vi "Read and Update Metadata.vi"(8 "error in (no error)":errorcluster, 11 "Update Metadata":bool) -> (0 "error out":errorcluster, 3 "Plugin Info":T1[](array[typedef]))   [LabVIEW 2021, in "CIFPluginLoader.lvclass"]
uses:
  CIFPluginLoader.lvclass
  typedef/trash_Discovered Plugin.ctl
  CIFCore/Common/Typedef/Version.ctl
  typedef/trash_Plugin Metadata.ctl
  CIFUtilities/CIFConfigurationFile/typedef/Location Type.ctl
  CIFUtilities/CIFConfigurationFile/CIF Configuration File Location.vi
  CIFPluginLoader.lvclass/CIFPluginLoader.ctl
  CIFUtilities/CIFConfigurationFile/CIF Configuration File.lvlib
  <vilib>/Utility/config.llb/NI_LVConfig.lvlib
  CIFCore/Common/CIFCoreCommon.lvlib
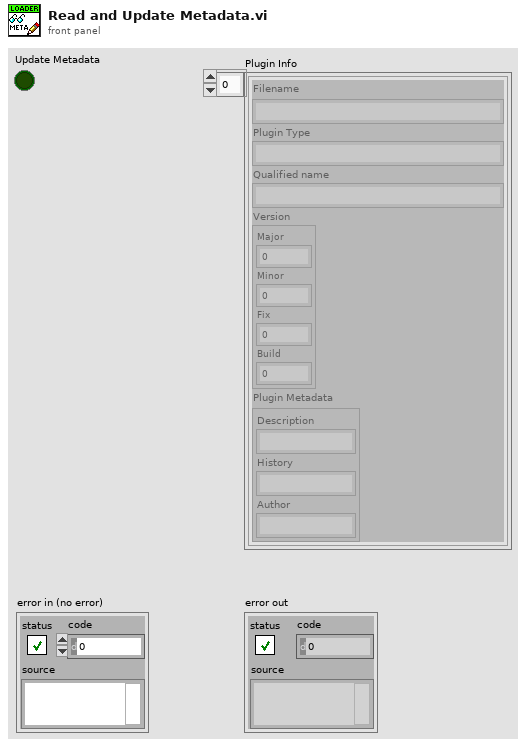
[diagram p1: front panel]
types:
  T1 = typedef "trash_Discovered Plugin.ctl" = cluster{"Filename":string, "Plugin Type":string, "Qualified name":string, "Version":T2, "Plugin Metadata":T3}
  T2 = typedef "CIFCoreCommon.lvlib/Version.ctl" = cluster{"Major":i32, "Minor":i32, "Fix":i32, "Build":i32}
  T3 = typedef "trash_Plugin Metadata.ctl" = cluster{"Description":string, "History":string, "Author":string}
  T4 = typedef "CIF Configuration File.lvlib/Location Type.ctl" = enum16{"Config File", "Manager", "Protos", "Plugins", "UI Plugins", "Logs", "Orchestrations"}
  T5 = typedef "NI_LVConfig.lvlib/Config Data RefNum.ctl" = refnum<k1>
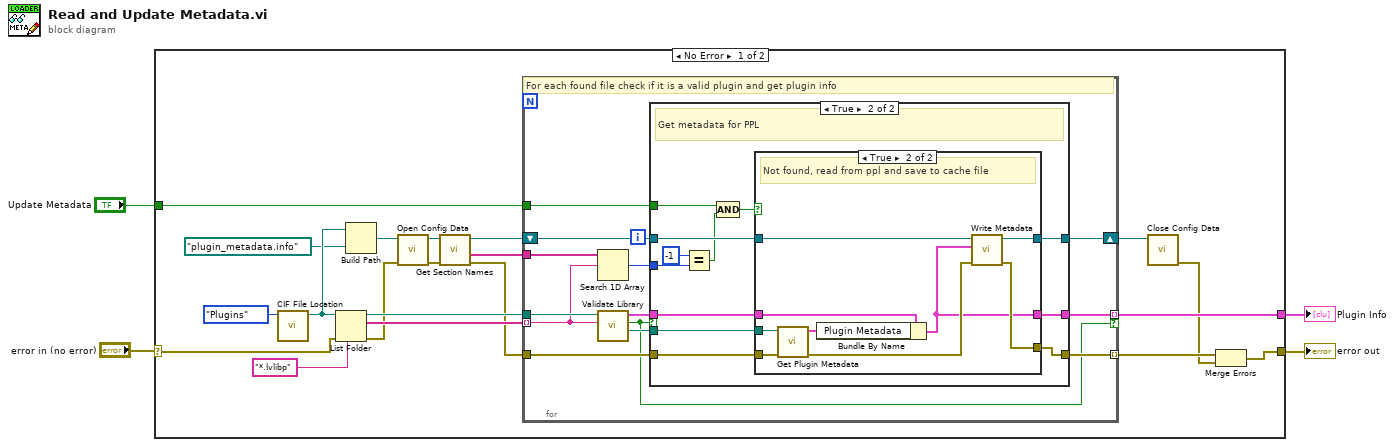
[diagram p0: block diagram]
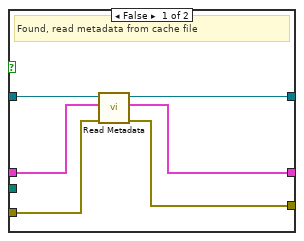
[diagram p3: hidden frame]
diagram:
  n1 = case shown="No Error" "error in (no error)" {
    selector: "error in (no error)" -> [w20 w68]
    tunnel: [w6 w68] -> w4
    tunnel: [w19 _] -> w2
    tunnel: "Update Metadata" -> [w5 _]
    frame No Error {
      n2 = call "CIF File Location.vi"("LocationType"=Location_Type."Plugins") -> ("Location"=w17:path)  [unwired: 10 in]
      n3 = List Folder(path=w17, pattern="*.lvlibp", error in=w20) -> (path out=w21:path, filenames=w22:string[], error out=w15:errorcluster)  [unwired: 1 in, 1 out]
      n4 = Build Path(base path=w17, name or relative path=path "plugin_metadata.info") -> (appended path=w18:path)
      n5 = call <vilib>:"Open Config Data.vi"("error in (no error)"=w15, "configuration file path"=w18) -> ("error out"=w12:errorcluster, "refnum"=w13:T5)  [unwired: 7 in, 1 out]
      n6 = call <vilib>:"Get Section Names.vi"("error in (no error)"=w12, "refnum"=w13) -> ("error out"=w10:errorcluster, "section names"=w9:string[], "refnum out"=w11:T5)  [unwired: 7 in]
      n7 = for {
        tunnel: w22 -> [w30] mode=indexing
        tunnel: w21 -> [w37]
        tunnel: [w35] -> w19 mode=indexing if=w26
        tunnel: w10 -> [w36]
        tunnel: [w34] -> w8 mode=indexing
        shift-right: [w32] -> w14
        shift-left: w11 -> [w33]
        tunnel: w9 -> [w31]
        tunnel: w5 -> [w25]
        # "For each found file check if it is a valid plugin and get plugin info"
        n8 = Search 1D Array(1D array=w31, element=w30) -> (index of element=w28:i32)  [unwired: 1 in]
        n9 = call "Validate Library.vi"("Filename"=w30, "path in"=w37) -> ("Full Path"=w27:path, "valid"=w26:bool, "Discovered Plugin"=w29:T1)  [unwired: 7 in]
        n10 = case shown="True" w26 {
          tunnel: w29 -> [w39 w52]
          tunnel: w27 -> [_ w51]
          tunnel: w36 -> [w40 w50]
          tunnel: [w39 w47] -> w35
          tunnel: [w40 w46] -> w34
          tunnel: w33 -> [w38 w49]
          tunnel: [w38 w48] -> w32
          tunnel: w28 -> [_ w45]
          tunnel: w25 -> [_ w43]
          frame False {
            # "Invalid"
          }
          frame True {
            # "Get metadata for PPL"
            n11 = Equal?(x=-1, y=w45) -> (x = y?=w42:bool)
            n12 = Compound Arithmetic op=AND(w43, w42) -> (w41:bool)
            n13 = case shown="True" w41 {
              tunnel: w52 -> [w57 w67]
              tunnel: w51 -> [_ w66]
              tunnel: w50 -> [w54 w64]
              tunnel: w49 -> [w58 w63]
              tunnel: [w55 w62] -> w48
              tunnel: [w56 w59] -> w47
              tunnel: [w53 w60] -> w46
              frame False {
                # "Found, read metadata from cache file"
                n14 = call "Read Metadata.vi"("error in (no error)"=w54, "Plugin Info in"=w57, "metadata ref in"=w58) -> ("error out"=w53:errorcluster, "Plugin Info out"=w56:T1, "metadata ref dup"=w55:T5)  [unwired: 6 in]
              }
              frame True {
                # "Not found, read from ppl and save to cache file"
                n15 = call "Get Plugin Metadata.vi"("error in (no error)"=w64, "Packed Library Path"=w66) -> ("error out"=w61:errorcluster, "Plugin Metadata"=w65:T3)  [unwired: 8 in]
                n16 = Bundle By Name(cluster=w67, "Plugin Metadata"=w65) -> (w59:T1)
                n17 = call "Write Metadata.vi"("error in (no error)"=w61, "Plugin Info"=w59, "metadata ref in"=w63) -> ("error out"=w60:errorcluster, "metadata ref dup"=w62:T5)  [unwired: 7 in]
              }
            }
          }
        }
      }
      n18 = call <vilib>:"Close Config Data.vi"("refnum"=w14) -> ("error out"=w7:errorcluster)  [unwired: 9 in, 1 out]
      n19 = Merge Errors(w8, w7) -> (w6:errorcluster)
    }
    frame Error {
    }
  }
  "error out" <- w4
  "Plugin Info" <- w2
